vi "(9) Move X (Stop and Scan) - Manual Control.vi"() -> ()   [LabVIEW 2020]
uses:
  <instrlib>/Arcus Ethernet Driver 1.0.0/ArcusEthernetComm/classes/Controller/_Controller.lvclass
panel:
  out "X Position (Steps)":string
  out "Y Position (Steps)":string
  out "Z Position (Steps)":string
  in  "Stop":bool
  in  "Direction":bool
  in  "X Desired Distance (mm)":dbl
  in  "error in (no error)":errorcluster
  in  "Stop and Scan":bool
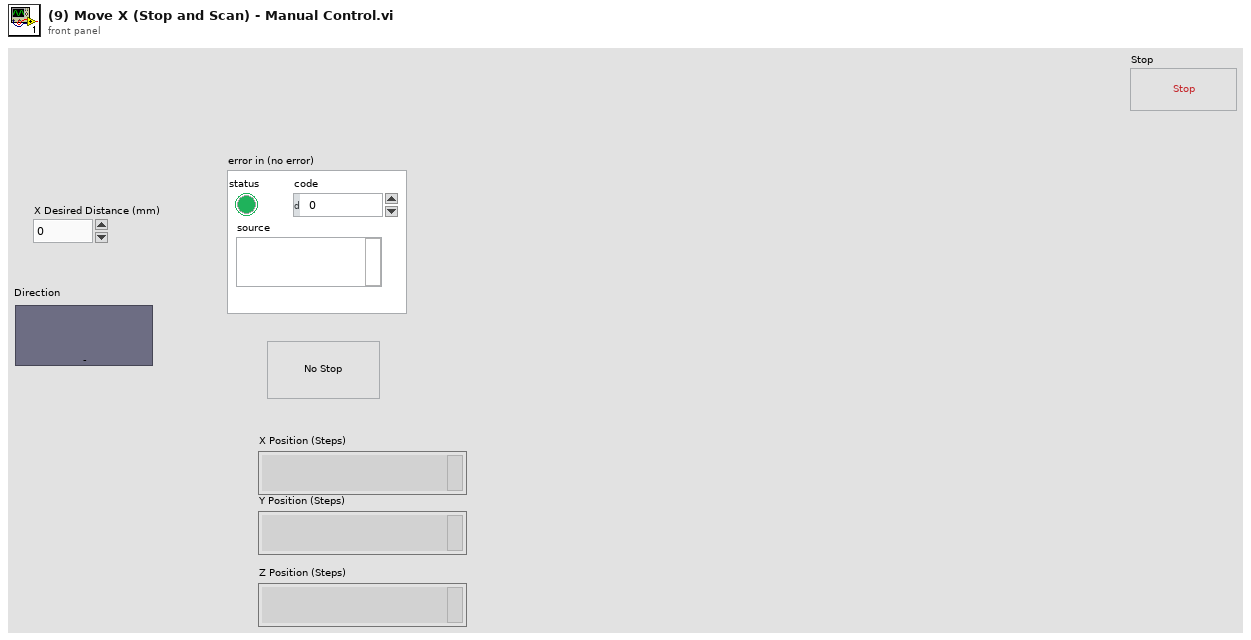
[diagram p1: front panel]
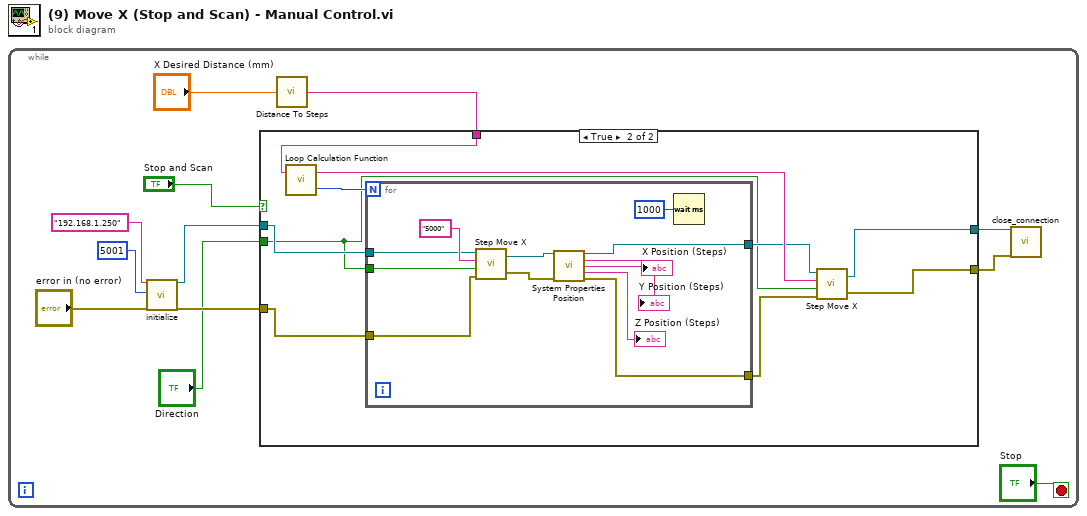
[diagram p0: block diagram]
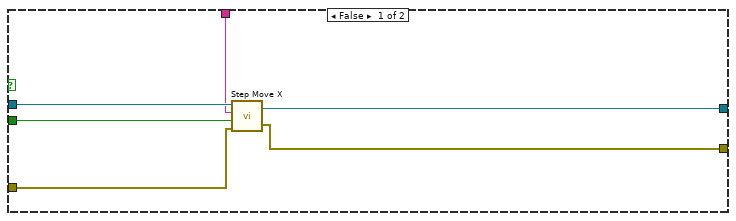
[diagram p2: hidden frame]
diagram:
  n1 = while {
    stop <- "Stop" stop-if-true
    n2 = call <instrlib>:"initialize.vi"("ip_address (in)"="192.168.1.250", "dev_port(def=5001)"=u16 5001, "error in (no error)"="error in (no error)") -> ("reference (out)"=w6:refnum<class "_Controller.lvclass">, "error out"=w5:errorcluster)  [unwired: 15 in]
    n3 = call "Distance To Steps.vi"("Desired Distance (mm)"="X Desired Distance (mm)") -> ("Number of Steps"=w4:string)
    n4 = case shown="True" "Stop and Scan" {
      tunnel: [w18 w22] -> w11
      tunnel: [w17 w21] -> w10
      tunnel: w6 -> [w16 w23]
      tunnel: w5 -> [w15 w24]
      tunnel: w4 -> [w14 w20]
      tunnel: "Direction" -> [w13 w19]
      frame False {
        n5 = call "Step Move X.vi"("error in (no error)"=w15, "Direction"=w13, "x steps"=w14, "reference (in)"=w16) -> ("error out"=w17:errorcluster, "reference (out)"=w18:refnum<class "_Controller.lvclass">)
      }
      frame True {
        n6 = call "Loop Calculation Function.vi"("Number of Steps"=w20) -> ("No. of Loops (-1)"=w25:i32, "Remainder"=w28:string)  [unwired: 1 in]
        n7 = for {
          N: w25 -> [_]
          tunnel: w23 -> [w34]
          tunnel: w24 -> [w33]
          tunnel: [w32] -> w27
          tunnel: [w31] -> w26
          tunnel: w19 -> [w30]
          n8 = call "Step Move X.vi"("error in (no error)"=w33, "Direction"=w30, "x steps"="5000" ("X Steps"), "reference (in)"=w34) -> ("error out"=w40:errorcluster, "reference (out)"=w36:refnum<class "_Controller.lvclass">)
          n9 = call "System Properties Position.vi"("reference (in)"=w36, "error in (no error)"=w40) -> ("reference (out)"=w31:refnum<class "_Controller.lvclass">, "X Position (Steps)"=→"X Position (Steps)":string, "Y Position (Steps)"=→"Y Position (Steps)":string, "Z Position (Steps)"=→"Z Position (Steps)":string, "error out"=w32:errorcluster)  [unwired: 9 in]
          n10 = Wait (ms)(milliseconds to wait=u32 1000) -> ()  [unwired: 1 out]
        }
        n11 = call "Step Move X.vi"("error in (no error)"=w27, "Direction"=w19, "x steps"=w28, "reference (in)"=w26) -> ("error out"=w21:errorcluster, "reference (out)"=w22:refnum<class "_Controller.lvclass">)
      }
    }
    n12 = call <instrlib>:"close_connection.vi"("reference (in)"=w11, "error in (no error)"=w10) -> ()  [unwired: 16 in, 2 out]
  }
